vi "Test_ConstructTransport_BadFormatString_Error.vi"(8 "error in (no error)":errorcluster, 11 "TestCase in":refnum<class "TestBooleanTextBinding.lvclass">) -> (0 "error out":errorcluster, 3 "TestCase out":refnum<class "TestBooleanTextBinding.lvclass">)   [LabVIEW 2017, in "TestBooleanTextBinding.lvclass"]
uses:
  TestBooleanTextBinding.lvclass
  Source/Concrete/BooleanTextBinding/BooleanTextBinding.lvclass/BooleanTextBinding.ctl
  <vilib>/Utility/error.llb/Error Cluster From Error Code.vi
  Source/Concrete/BooleanTextBinding/BooleanTextBinding.lvclass
panel:
  out "Return Error":errorcluster
  in  "OK Button":bool
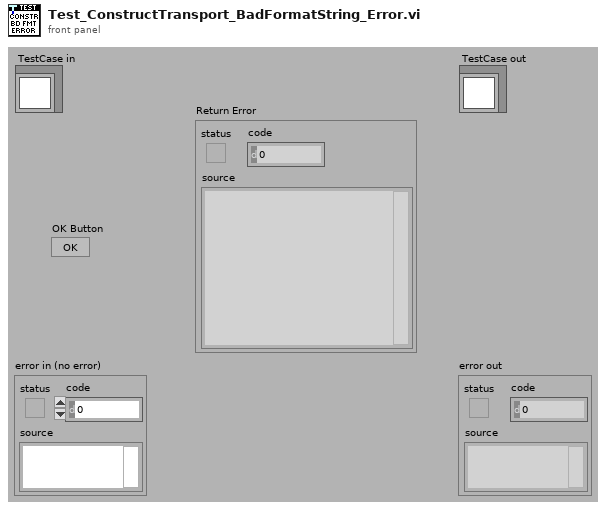
[diagram p1: front panel]
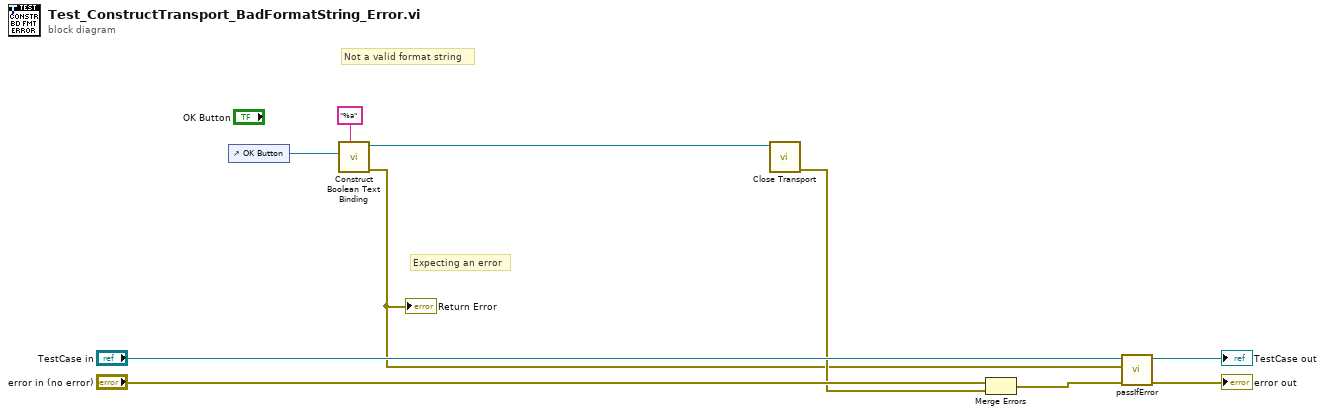
[diagram p0: block diagram]
diagram:
  # "Expecting an error"
  # "Not a valid format string"
  n1 = control-ref of="OK Button"() -> (w5:refnum<vi>)
  n2 = call "Construct Boolean Text Binding.vi"("Format String"="%a", "Bool Refnum"=w5) -> ("error out"=w1:errorcluster, "BooleanTextBinding"=w2:refnum<class "BooleanTextBinding.lvclass">)  [unwired: 8 in]
  "Return Error" <- w1
  n3 = call-dynamic "Close Transport.vi"("ITransport in"=w2) -> ("error out"=w4:errorcluster)  [unwired: 10 in]
  n4 = Merge Errors("error in (no error)", w4) -> (w6:errorcluster)
  n5 = call-dynamic "passIfError.vi"("error in (no error)"=w6, "error"=w1, "TestCase in"="TestCase in") -> ("error out"=→"error out":errorcluster, "TestCase out"=→"TestCase out":refnum<class "TestBooleanTextBinding.lvclass">)  [unwired: 7 in]
